vi "Read Enabled Values.vi"(8 "error in (no error)":errorcluster, 11 "NI Digital in":refnum<class "String Out.lvclass">) -> (0 "error out":errorcluster, 2 "Data Values":dbl[](array[numeric]), 3 "NI Digital out":refnum<class "String Out.lvclass">)   [LabVIEW 2018, in "String Out.lvclass"]
uses:
  String Out.lvclass
  String Out.lvclass/String Out.ctl
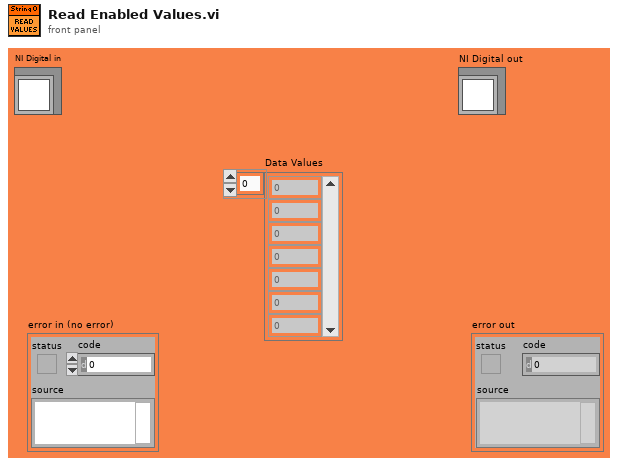
[diagram p1: front panel]
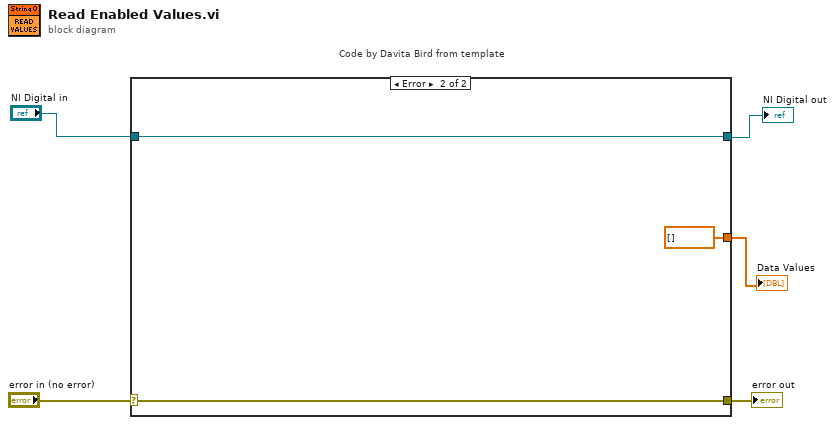
[diagram p0: block diagram]
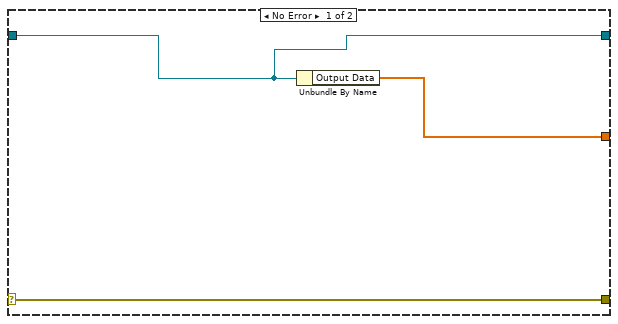
[diagram p2: hidden frame]
diagram:
  n1 = case "Code by Davita Bird from template" shown="Error" "error in (no error)" {
    selector: "error in (no error)" -> [w8 w11]
    tunnel: [w8 w11] -> w4
    tunnel: [w7 w10] -> w1
    tunnel: "NI Digital in" -> [w7 w10]
    tunnel: [w6 dbl[] [] ("array type (2D Dbl)")] -> w3
    frame No Error {
      n2 = Unbundle By Name(w7) -> ("Output Data"=w6:dbl[])
    }
    frame Error {
    }
  }
  "error out" <- w4
  "Data Values" <- w3
  "NI Digital out" <- w1
